vi "Tester_v01.vi"() -> ()   [LabVIEW 2015]
uses:
  <vilib>/LabVIEW Interface for Arduino/Type Defs/Connection Type.ctl
  <vilib>/LabVIEW Interface for Arduino/Type Defs/Pin Mode.ctl
  <vilib>/LabVIEW Interface for Arduino/Type Defs/Board Type.ctl
  <vilib>/LabVIEW Interface for Arduino/LabVIEW Interface for Arduino.lvlib
panel:
  out "Tab Control":T1(tab)
  out "?":string
  in  "Exit the program":bool
  in  "Start Test":bool
  in  "Next Button 2":bool
  out "String 2":string
  in  "Next Button 3":bool
  out "String 3":string
  in  "stop 3":bool
  in  "Next Button 4":bool
  out "String 4":string
  in  "stop K1":bool
  out "Error K1":string
  out "Progress Bar":u8(slide) scale=0.0..100.0
  out "String 5":string
  in  "stop Error":bool
  out "Last  Message 2":string
  in  "Complete":bool
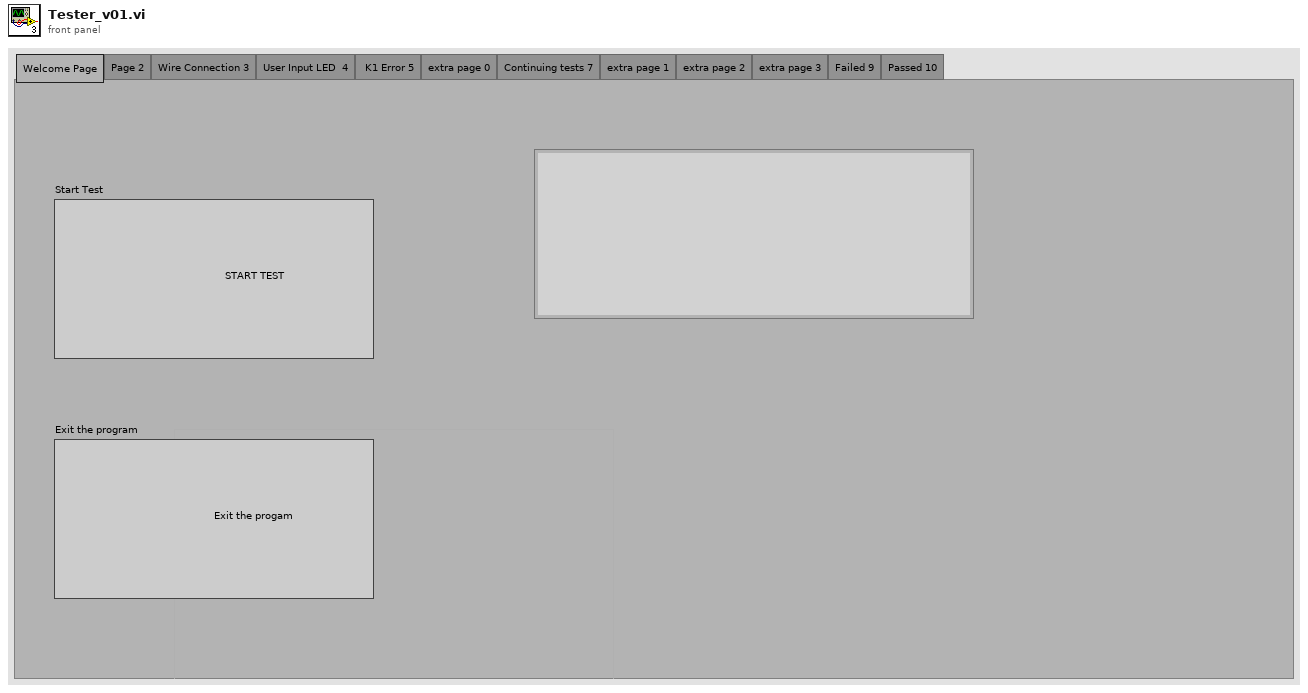
[diagram p1: front panel]
types:
  T1 = enum32{"Welcome Page", "Page 2", "Wire Connection 3", "User Input LED  4", " K1 Error 5", "extra page 0", "Continuing tests 7", "extra page 1", "extra page 2", "extra page 3", "Failed 9", "Passed 10"}
  T2 = enum8{"Enabled", "Disabled", "Disabled and Grayed Out"}
  T3 = typedef "LabVIEW Interface for Arduino.lvlib/Pin Mode.ctl" = enum8{"Input", "Output"}
  T4 = typedef "LabVIEW Interface for Arduino.lvlib/Connection Type.ctl" = enum8{"USB / Serial", "XBEE", "BlueSmirf (Bluetooth)"}
  T5 = typedef "LabVIEW Interface for Arduino.lvlib/Board Type.ctl" = enum16{"Uno", "Dimuelanove w/Atmega 328", "Mega 2560"}
  T6 = enum32{"Page 1", "Page 2", "Page 3", "Page 4", "Page 5", "Page 6", "Page 7", "Page 8", "Page 9"}
  T7 = typedef "LabVIEW Interface for Arduino.lvlib/Arduino Resource.ctl" = cluster{"VISA resource":refnum<visa-resource-name>, "Board Type":T5, "Connection Type":enum8{"USB / Serial"}, "Bytes Per Packet (15)":u8}
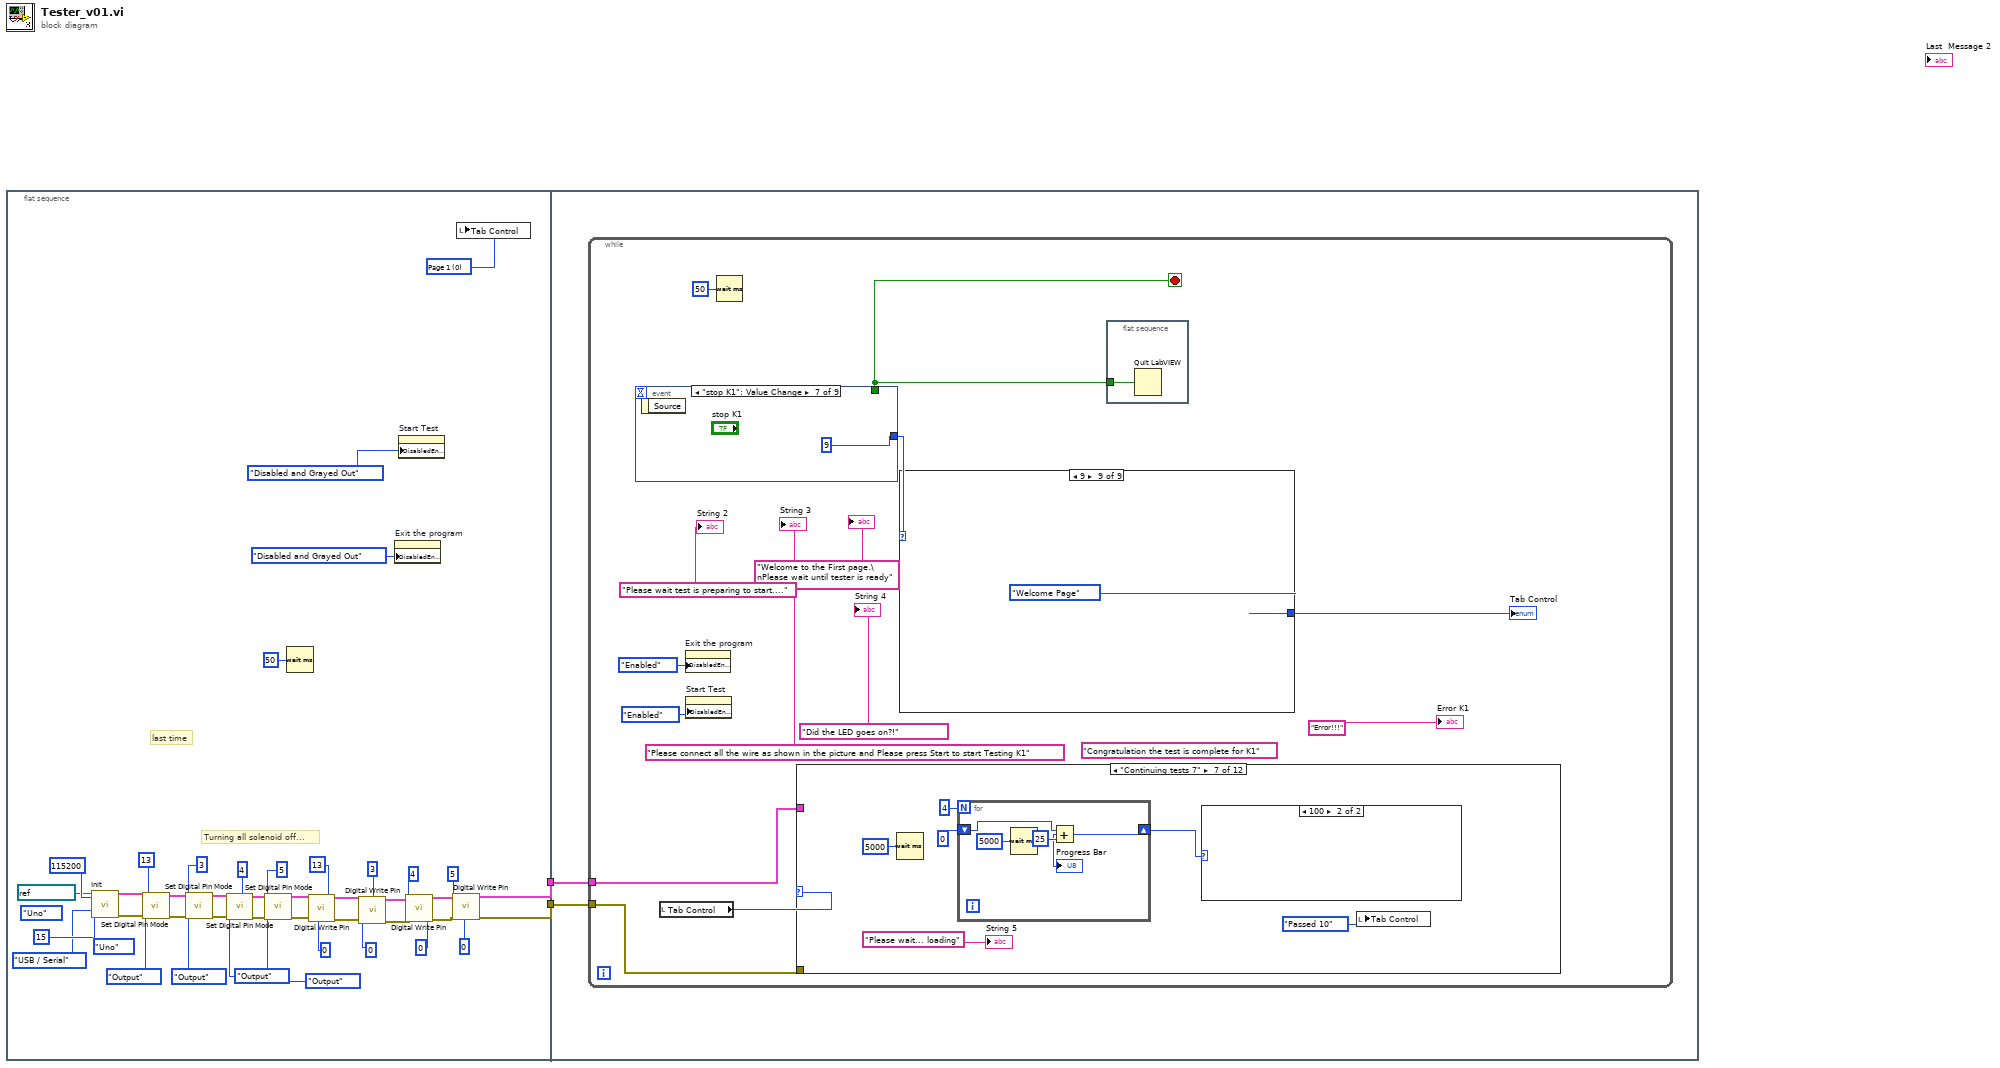
[diagram p0: block diagram]
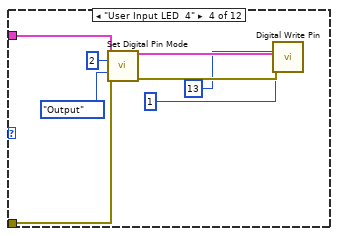
[diagram p5: hidden frame]
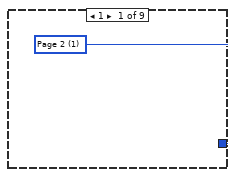
[diagram p14: hidden frame]
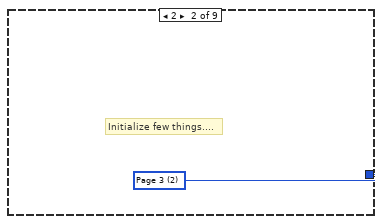
[diagram p15: hidden frame]
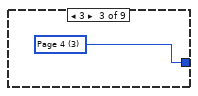
[diagram p16: hidden frame]
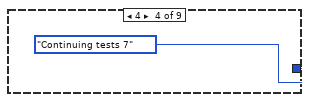
[diagram p17: hidden frame]
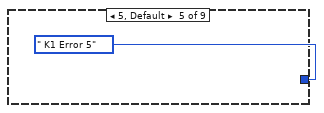
[diagram p18: hidden frame]
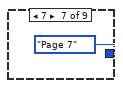
[diagram p20: hidden frame]
diagram:
  n1 = flat-sequence {
    tunnel: [w15] -> w2
    tunnel: [w14] -> w1
    tunnel: w2 -> [w47]
    tunnel: w1 -> [w46]
    frame #0 {
      (unwired) Board_Type."Uno" ("Board Type (Uno)")
      w45 = u16 0 items=["Page 1"]
      # "last time"
      # "Turning all solenoid off..."
      n2 = call <vilib>:"Init.vi"("VISA resource"=refnum<visa-resource-name> "COM73", "Baud Rate (115200)"=u32 115200, "Board Type (Uno)"=Board_Type."Uno", "Bytes Per Packet (15)"=u32 15, "Connection Type (USB/Serial)"=Connection_Type."USB / Serial") -> ("Arduino Resource"=w40:T7, "error out"=w39:errorcluster)  [unwired: 13 in]
      n3 = call <vilib>:"Set Digital Pin Mode.vi"("Arduino Resource"=w40, "Digital I/O Pin"=u8 13, "Pin Mode (Input)"=Pin_Mode."Output", "error in"=w39) -> ("Arduino Resource"=w38:T7, "error out"=w37:errorcluster)  [unwired: 10 in]
      n4 = call <vilib>:"Set Digital Pin Mode.vi"("Arduino Resource"=w38, "Digital I/O Pin"=u8 3, "Pin Mode (Input)"=Pin_Mode."Output", "error in"=w37) -> ("Arduino Resource"=w36:T7, "error out"=w35:errorcluster)  [unwired: 10 in]
      n5 = call <vilib>:"Set Digital Pin Mode.vi"("Arduino Resource"=w36, "Digital I/O Pin"=u8 4, "Pin Mode (Input)"=Pin_Mode."Output", "error in"=w35) -> ("Arduino Resource"=w34:T7, "error out"=w33:errorcluster)  [unwired: 10 in]
      n6 = call <vilib>:"Set Digital Pin Mode.vi"("Arduino Resource"=w34, "Digital I/O Pin"=u8 5, "Pin Mode (Input)"=Pin_Mode."Output", "error in"=w33) -> ("Arduino Resource"=w23:T7, "error out"=w22:errorcluster)  [unwired: 10 in]
      n7 = Wait (ms)(milliseconds to wait=u32 50) -> ()  [unwired: 1 out]
      n8 = call <vilib>:"Digital Write Pin.vi"("Arduino Resource"=w23, "Digital I/O Pin (0)"=u8 13 ("Digital I/O Pin"), "Value (0)"=u8 0, "error in"=w22) -> ("Arduino Resource"=w21:T7, "error out"=w20:errorcluster)  [unwired: 10 in]
      n9 = call <vilib>:"Digital Write Pin.vi"("Arduino Resource"=w21, "Digital I/O Pin (0)"=u8 3 ("Digital I/O Pin"), "Value (0)"=u8 0, "error in"=w20) -> ("Arduino Resource"=w19:T7, "error out"=w18:errorcluster)  [unwired: 10 in]
      n10 = property on="Exit the program" class="Bool"("DisabledEnum"=T2."Disabled and Grayed Out" ("Disabled")) -> ()  [unwired: 2 in, 2 out]
      n11 = property on="Start Test" class="Bool"("DisabledEnum"=T2."Disabled and Grayed Out" ("Disabled")) -> ()  [unwired: 2 in, 2 out]
      n12 = call <vilib>:"Digital Write Pin.vi"("Arduino Resource"=w19, "Digital I/O Pin (0)"=u8 4 ("Digital I/O Pin"), "Value (0)"=u8 0, "error in"=w18) -> ("Arduino Resource"=w17:T7, "error out"=w16:errorcluster)  [unwired: 10 in]
      n13 = call <vilib>:"Digital Write Pin.vi"("Arduino Resource"=w17, "Digital I/O Pin (0)"=u8 5 ("Digital I/O Pin"), "Value (0)"=u8 0, "error in"=w16) -> ("Arduino Resource"=w15:T7, "error out"=w14:errorcluster)  [unwired: 10 in]
      n14 = local write "Tab Control"(w45) -> ()
    }
    frame #1 {
      n15 = while {
        tunnel: w47 -> [w51]
        tunnel: w46 -> [w50]
        stop <- w56 stop-if-true
        (unwired) "Congratulation the test is complete for K1" ("Last  Message")
        n16 = event shown="[6] \"stop K1\": Value Change" {
          selector: _ -> [_ _ _ _ _ _ _ _ _]
          dyn-events: _ -> [_ _ _ _ _ _ _ _ _]
          timeout: _ -> [_ _ _ _ _ _ _ _ _]
          tunnel: [1 _ 2 3 4 5 9 7 9] -> w60
          tunnel: [_ "Exit the program" _ _ _ _ _ _ _] -> w56
          event "Start Test": Value Change {
            n17 = event-data() -> ()  [unwired: 1 in, 1 out]
          }
          event "Exit the program": Value Change {
            n18 = event-data() -> ()  [unwired: 1 in, 1 out]
          }
          event "Next Button 2": Value Change {
            n19 = event-data() -> ()  [unwired: 1 in, 1 out]
          }
          event "Next Button 3": Value Change {
            n20 = event-data() -> ()  [unwired: 1 in, 1 out]
          }
          event "Next Button 4": Value Change {
            n21 = event-data() -> ()  [unwired: 1 in, 1 out]
          }
          event "stop 3": Value Change {
            n22 = event-data() -> ()  [unwired: 1 in, 1 out]
          }
          event "stop K1": Value Change {
            n23 = event-data() -> ()  [unwired: 1 in, 1 out]
          }
          event "stop Error": Value Change {
            n24 = event-data() -> ()  [unwired: 1 in, 5 out]
          }
          event "Complete": Value Change {
            n25 = event-data() -> ()  [unwired: 1 in, 5 out]
          }
        }
        n26 = local read "Tab Control"() -> (w52:T1)
        n27 = property on="Exit the program" class="Bool"("DisabledEnum"=T2."Enabled" ("Disabled")) -> ()  [unwired: 2 in, 2 out]
        n28 = property on="Start Test" class="Bool"("DisabledEnum"=T2."Enabled" ("Disabled")) -> ()  [unwired: 2 in, 2 out]
        n29 = Wait (ms)(milliseconds to wait=u32 50) -> ()  [unwired: 1 out]
        n30 = case shown="\"Continuing tests 7\"" w52 {
          tunnel: w51 -> [_ _ _ w69 _ _ _ _ _ _ _ _]
          tunnel: w50 -> [_ _ _ w68 _ _ _ _ _ _ _ _]
          frame "Welcome Page", Default {
          }
          frame "Page 2" {
          }
          frame "Wire Connection 3" {
          }
          frame "User Input LED  4" {
            n31 = call <vilib>:"Set Digital Pin Mode.vi"("Arduino Resource"=w69, "Digital I/O Pin"=u8 2, "Pin Mode (Input)"=Pin_Mode."Output", "error in"=w68) -> ("Arduino Resource"=w65:T7, "error out"=w64:errorcluster)  [unwired: 10 in]
            n32 = call <vilib>:"Digital Write Pin.vi"("Arduino Resource"=w65, "Digital I/O Pin (0)"=u8 13, "Value (0)"=u8 1, "error in"=w64) -> ()  [unwired: 10 in, 2 out]
          }
          frame " K1 Error 5" {
          }
          frame "extra page 0" {
          }
          frame "Continuing tests 7" {
            n33 = Wait (ms)(milliseconds to wait=u32 5000) -> ()  [unwired: 1 out]
            n34 = for {
              N: 4 -> [_]
              shift-right: [w76] -> w71
              shift-left: 0 -> [w77]
              n35 = Wait (ms)(milliseconds to wait=u32 5000) -> ()  [unwired: 1 out]
              n36 = Add(x=w77, y=25) -> (x+y=w76:i32)
              "Progress Bar" <- w76
            }
            n37 = case shown="100" w71 {
              frame 0, Default {
              }
              frame 100 {
              }
            }
            n38 = local write "Tab Control"(T1."Passed 10" ("Tab Control")) -> ()
            "String 5" <- "Please wait... loading" ("String 5")
          }
          frame "extra page 1" {
          }
          frame "extra page 2" {
          }
          frame "extra page 3" {
          }
          frame "Failed 9" {
          }
          frame "Passed 10" {
          }
        }
        n39 = case shown="9" w60 {
          tunnel: [w80 w81 w82 T1."Continuing tests 7" ("Tab Control") T1." K1 Error 5" ("Tab Control") _ T6."Page 7" ("Tab Control") T6."Page 7" ("Tab Control") T1."Welcome Page" ("Tab Control")] -> w54
          frame 1 {
            w80 = u16 1 items=["Page 1", "Page 2", "Page 3"]
          }
          frame 2 {
            w81 = u16 2 items=["Page 1", "Page 2", "Page 3", "Page 4"]
            # "Initialize few things...."
          }
          frame 3 {
            w82 = u16 3 items=["Page 1", "Page 2", "Page 3", "Page 4", "Page 5"]
          }
          frame 4 {
          }
          frame 5, Default {
          }
          frame 6 {
          }
          frame 7 {
          }
          frame 8 {
          }
          frame 9 {
          }
        }
        "Tab Control" <- w54
        n40 = flat-sequence {
          tunnel: w56 -> [w97]
          frame #0 {
            n41 = Quit LabVIEW(quit? (T)=w97) -> ()
          }
        }
        "?" <- "Welcome to the First page.\nPlease wait until tester is ready"
        "String 2" <- "Please wait test is preparing to start...."
        "String 3" <- "Please connect all the wire as shown in the picture and Please press Start to start Testing K1"
        "String 4" <- "Did the LED goes on?!"
        "Error K1" <- "Error!!!" ("Error")
      }
    }
  }
